vi "WriteFGVError.vi"(8 "error in (no error)":errorcluster, 10 "0Cv/1St":i32, 11 "AI in":refnum<class "AI.lvclass">) -> (0 "error out":errorcluster, 3 "AI out":refnum<class "AI.lvclass">)   [LabVIEW 2019, in "AI.lvclass"]
uses:
  AI.lvclass
  Ctrl/Auto Inspection Data Name.ctl
  Ctrl/Auto Inspection Station Name2.ctl
  c34c7080-bac7-4536-9648-5da41f0892c6.vi
  <vilib>/JDP Science/JSONtext/Variant to JSON Text.vi
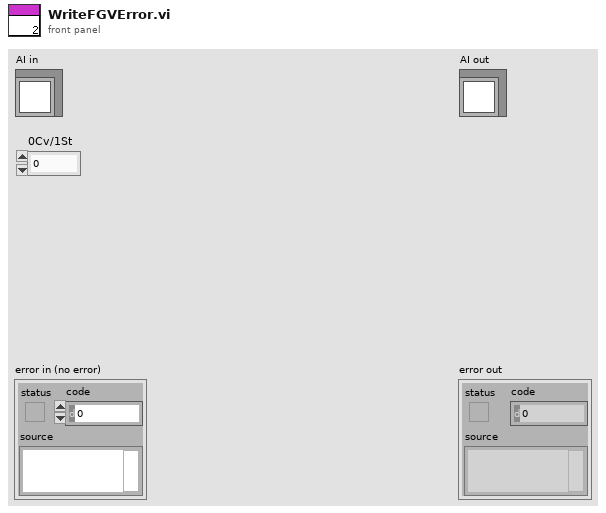
[diagram p1: front panel]
types:
  T1 = typedef "Auto Inspection Data Name.ctl" = enum16{"LocalRun", "ItemSN(TimeCode)", "CurrentAction", "Error", "Data", "OKNG", "電壓值", "電壓值判斷", "電流值", "電流值判斷", "Laser1 Data", "Laser2 Data", "Laser OKNG", "StationNO"}
  T2 = typedef "Auto Inspection Station Name2.ctl" = enum16{"S1Barcode", "S2Measure", "S3Measure", "S4Measure", "S5Measure", "S11_LaserCheck", "S8_Vision AI"}
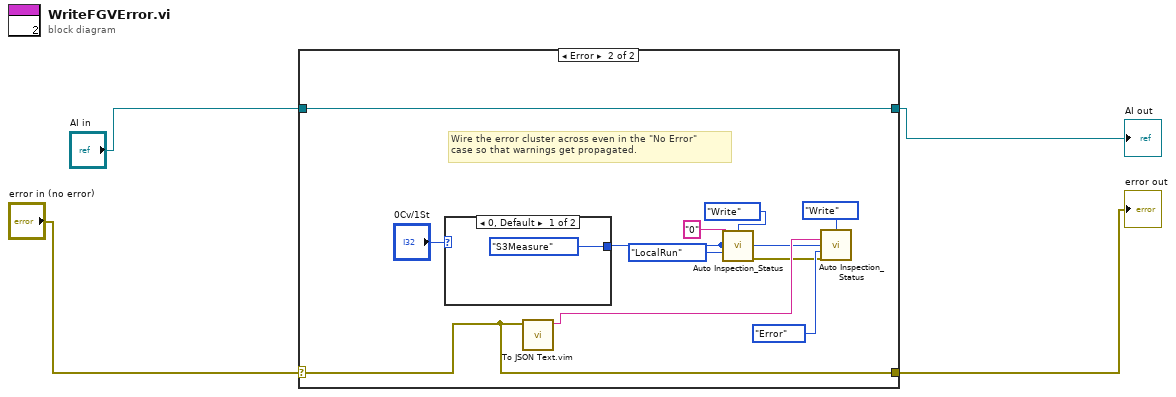
[diagram p0: block diagram]
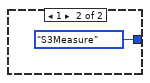
[diagram p3: hidden frame]
diagram:
  n1 = case shown="Error" "error in (no error)" {
    selector: "error in (no error)" -> [w6 w12]
    tunnel: [w6 w12] -> w1
    tunnel: [w5 w17] -> w2
    tunnel: "AI in" -> [w5 w17]
    frame No Error {
    }
    frame Error {
      # "Wire the error cluster across even in the \"No Error\"\ncase so that warnings get propagated."
      n2 = case shown="0, Default" "0Cv/1St" {
        tunnel: [Auto_Inspection_Station_Name2."S3Measure" ("Station") Auto_Inspection_Station_Name2."S3Measure" ("Station")] -> w10
        frame 0, Default {
        }
        frame 1 {
        }
      }
      n3 = call "To JSON Text.vim"("Anything"=w12) -> ("<JSON>"=w13:string)  [unwired: 9 in, 1 out]
      n4 = call "Auto Inspection_Status.vi"("Action"=enum16{"Initial", "Write", "Read"}."Write", "DataIn"="0", "Station"=w10, "Data"=Auto_Inspection_Data_Name."LocalRun") -> ("error out"=w9:errorcluster)  [unwired: 9 in, 2 out]
      n5 = call "Auto Inspection_Status.vi"("Action"=enum16{"Initial", "Write", "Read"}."Write", "DataIn"=w13, "Station"=w10, "Data"=Auto_Inspection_Data_Name."Error", "error in"=w9) -> ()  [unwired: 8 in, 3 out]
    }
  }
  "error out" <- w1
  "AI out" <- w2
